vi "Write 0D U16.vi"(8 "error in (no error)":errorcluster, 9 "offset (0)":u64 format="%d bytes", 10 "value in":u16, 11 "Buffer in":refnum<class "Buffer.lvclass">) -> (0 "error out":errorcluster, 1 "offset out":u64 format="%d bytes", 2 "value out":u16, 3 "Buffer out":refnum<class "Buffer.lvclass">)   [LabVIEW 2017, in "DSF Core.lvlib" / "Buffer.lvclass"]
uses:
  Buffer.lvclass
  C:/Program Files (x86)/National Instruments/LabVIEW 2017/vi.lib/NI/Memory Manager/Classes/Pointer/Memory.Pointer.lvclass
  <vilib>/NI/Memory Manager/Classes/Pointer/Memory.Pointer.lvclass/Memory.Pointer.ctl
  <vilib>/NI/Memory Manager/Classes/Pointer/Memory.Pointer.Write.0D.U16.vi
  <vilib>/NI/Memory Manager/Classes/Pointer/Memory.Pointer.Write.No Check.0D.U16.vi
  <vilib>/NI/Memory Manager/Classes/Pointer/Memory.Pointer.Parameter Check.Null Pointer.vi
  <vilib>/NI/Memory Manager/Classes/Pointer/Memory.Pointer.Parameter Check.Subset.vi
  <vilib>/NI/Memory Manager/Classes/Pointer/Memory.Pointer.Get Address.vi
  <vilib>/NI/Memory Manager/Classes/Pointer/Memory.Pointer.Errors.vi
  <vilib>/NI/Memory Manager/Classes/Pointer/Memory.Pointer.Errors.Null Pointer.vi
  <vilib>/NI/Memory Manager/Classes/Pointer/Memory.Pointer.Errors.Out of Bounds.vi
  <vilib>/NI/Memory Manager/Classes/Pointer/Memory.Pointer.Get Size.vi
  <vilib>/NI/Memory Manager/Classes/Pointer/Memory.Pointer.Errors.Create Error.vi
  <vilib>/NI/Memory Manager/VIs/Source.Write.String.vi
  <vilib>/NI/Memory Manager/Classes/Pointer/Memory.Pointer.Errors.Write Pointer Size.vi
  <vilib>/NI/Memory Manager/VIs/Source.Write.Scalar.Base10.vi
  <vilib>/NI/Memory Manager/VIs/Source.Write.Scalar.Base10 (U64).vi
  <vilib>/NI/Memory Manager/VIs/New Error Cluster Constant.vi
  <vilib>/NI/Memory Manager/VIs/New Error Cluster Constant (512B).vi
  <vilib>/NI/Memory Manager/VIs/Error Cluster.Set Status.vi
  <vilib>/NI/Memory Manager/VIs/Error Cluster.Set Code.vi
  <vilib>/NI/Memory Manager/VIs/Error Cluster.Set VI Source.vi
  <vilib>/NI/Memory Manager/Constants/Memory.Constants.vi
  <vilib>/NI/Memory Manager/Constants/Memory.Constants.Library Name.vi
  <vilib>/NI/Memory Manager/Classes/Pointer/Memory.Pointer.Errors.Get Info.vi
  <vilib>/NI/Memory Manager/Classes/Pointer/Memory.Pointer.lvclass
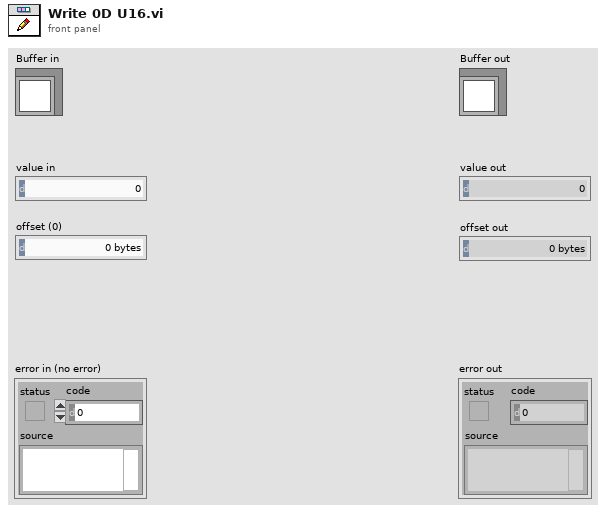
[diagram p1: front panel]
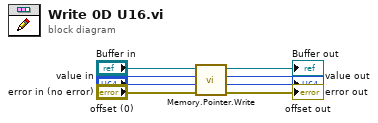
[diagram p0: block diagram]
diagram:
  n1 = call-poly <vilib>:"Memory.Pointer.Write.vi"("error in (no error)"="error in (no error)", "offset (0)"="offset (0)", "value"="value in", "Pointer in"="Buffer in") -> ("error out"=→"error out":errorcluster, "offset out"=→"offset out":u64, "value"=→"value out":u16, "Pointer out"=→"Buffer out":refnum<class "Buffer.lvclass">)  [unwired: 4 in]
